vi "InitDataSets.vi"(8 "error in (no error)":errorcluster, 10 "registry":T1, 11 "dataevent":T6) -> (0 "error out":errorcluster, 2 "datasetIds":variant, 3 "datasets":T7[](array[typedef]))   [LabVIEW 2017, in "EmsaDataEventCreator.lvlib"]
uses:
  <vilib>/addons/InsightCM/Devices/Shared/Emsa/EmsaDataEventCreator/EmsaDataEventCreator.lvlib
  <vilib>/addons/InsightCM/Devices/Shared/Common/DataEvent/controls/DataSet.ctl
  <vilib>/addons/InsightCM/MessageBus/Base/controls/DataSetMetadata.ctl
  <vilib>/addons/InsightCM/MessageBus/Base/controls/KeyValuePair.ctl
  <vilib>/addons/InsightCM/MessageBus/Base/controls/DataEvent.ctl
  <vilib>/addons/InsightCM/Devices/Shared/Emsa/EmsaDataEventCreator/controls/Registry.ctl
  <vilib>/addons/InsightCM/Devices/Shared/Emsa/EmsaDataEventCreator/controls/Registry_Sweep.ctl
  <vilib>/addons/InsightCM/Devices/Shared/Common/DataEvent/controls/DataSetType.ctl
  <vilib>/addons/InsightCM/Devices/Shared/Common/DataEventCreator/controls/Registry_Trend.ctl
  <vilib>/addons/InsightCM/Devices/Shared/Common/DataEvent/DataEvent.lvlib
  <vilib>/addons/InsightCM/SRP/SRP.lvlib
  <vilib>/addons/InsightCM/Devices/Shared/Common/DataEventCreator/DataEventCreator.lvlib
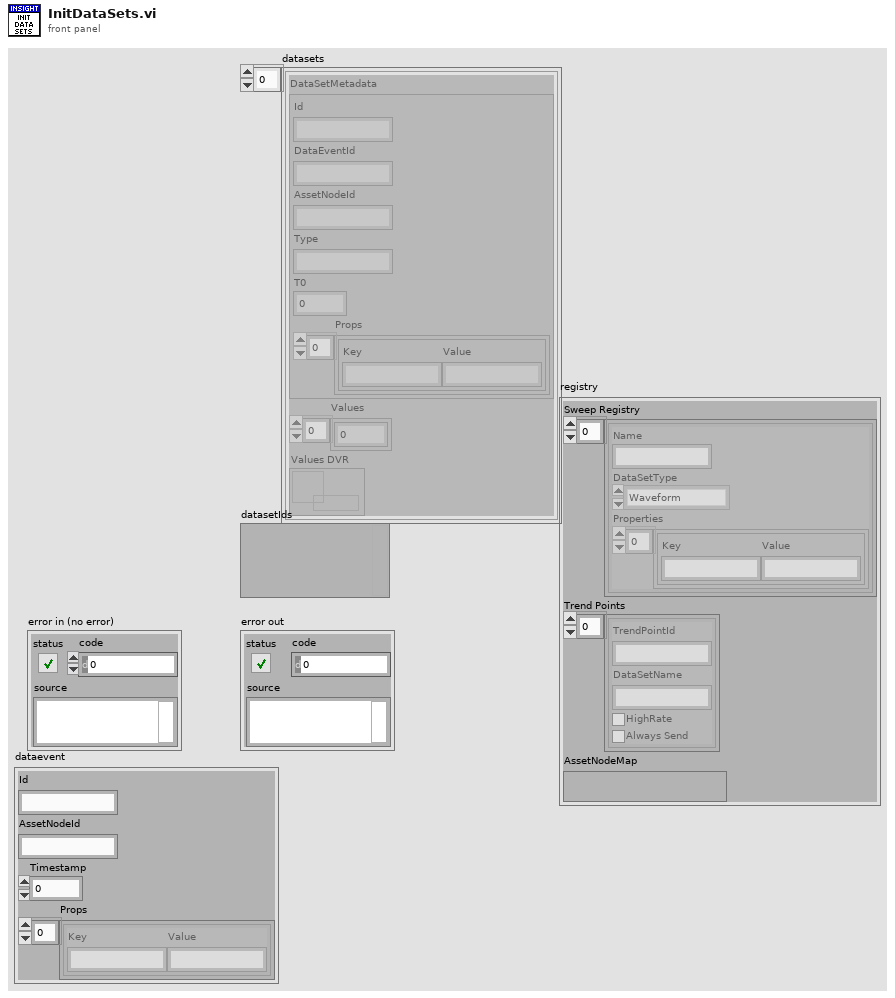
[diagram p1: front panel]
types:
  T1 = typedef "EmsaDataEventCreator.lvlib/Registry.ctl" = cluster{"Sweep Registry":T2[], "Trend Points":T5[], "AssetNodeMap":variant}
  T2 = typedef "EmsaDataEventCreator.lvlib/Registry_Sweep.ctl" = cluster{"Name":string, "DataSetType":T3, "Properties":T4[]}
  T3 = typedef "DataEvent.lvlib/DataSetType.ctl" = enum16{"Waveform", "SpeedProfile", "ThermalImage", "EmsaSweep"}
  T4 = typedef "KeyValuePair.ctl" = cluster{"Key":string, "Value":string}
  T5 = typedef "DataEventCreator.lvlib/Registry_Trend.ctl" = cluster{"TrendPointId":string, "DataSetName":string, "HighRate":bool, "Always Send":bool}
  T6 = typedef "DataEvent.ctl" = cluster{"Id":string, "AssetNodeId":string, "Timestamp":i64, "Props":T4[]}
  T7 = typedef "DataEvent.lvlib/DataSet.ctl" = cluster{"DataSetMetadata":T8, "Values":sgl[], "Values DVR":refnum<data-value>}
  T8 = typedef "DataSetMetadata.ctl" = cluster{"Id":string, "DataEventId":string, "AssetNodeId":string, "Type":string, "T0":i64, "Props":T4[]}
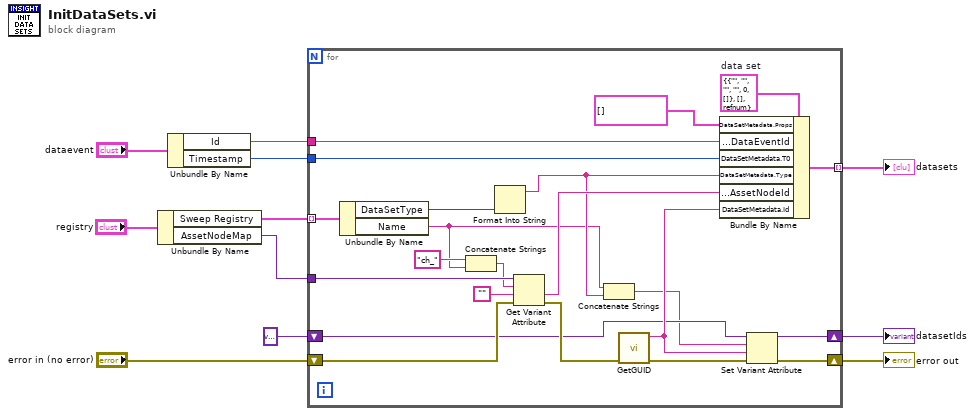
[diagram p0: block diagram]
diagram:
  n1 = Unbundle By Name("registry") -> ("Sweep Registry"=w4:T2[], "AssetNodeMap"=w5:variant)
  n2 = Unbundle By Name("dataevent") -> ("Id"=w8:string, "Timestamp"=w7:i64)
  n3 = for {
    tunnel: w5 -> [w27]
    shift-right: [w32] -> w2
    shift-left: variant -> [w21]
    shift-right: [w31] -> w1
    shift-left: "error in (no error)" -> [w29]
    tunnel: [w23] -> w3 mode=indexing
    tunnel: w8 -> [w20]
    tunnel: w7 -> [w19]
    tunnel: w4 -> [w16] mode=indexing
    w25 = T7 {"DataSetMetadata"={"Id"="", "DataEventId"="", "AssetNodeId"="", "Type"="", "T0"=0, "Props"=[]}, "Values"=[], "Values DVR"=refnum}  # data set
    n4 = Unbundle By Name(w16) -> ("DataSetType"=w30:T3, "Name"=w13:string)
    n5 = Concatenate Strings("ch_" ("string"), w13) -> (w12:string)
    n6 = Format Into String(w30) -> (resulting string=w17:string)  [unwired: 3 in, 1 out]
    n7 = Get Variant Attribute(Variant=w27, name=w12, default value (empty Variant)="", error in=w29) -> (value=w24:string, error out=w28:errorcluster)  [unwired: 2 out]
    n8 = Concatenate Strings(w13, w17) -> (w18:string)
    n9 = call <vilib>:"GetGUID.vi"("error in (no error)"=w28) -> ("error out"=w33:errorcluster, "GUID"=w22:string)  [unwired: 9 in]
    n10 = Bundle By Name(cluster=w25, "DataSetMetadata.Props"=T4[] [] ("key value pairs"), "DataSetMetadata.DataEventId"=w20, "DataSetMetadata.T0"=w19, "DataSetMetadata.Type"=w17, "DataSetMetadata.AssetNodeId"=w24, "DataSetMetadata.Id"=w22) -> (w23:T7)
    n11 = Set Variant Attribute(Variant=w21, name=w18, value=w22, error in=w33) -> (Variant out=w32:variant, error out=w31:errorcluster)  [unwired: 1 out]
  }
  "datasets" <- w3
  "error out" <- w1
  "datasetIds" <- w2
